vi "Periodic Tasks.vi"(11 "error in":errorcluster) -> ()   [LabVIEW 2012]
doc: "This VI runs in parallel to other tasks. It can contain as many user-defined periodic loops as you need. These can carry out PID or other sorts of timed response."
uses:
  <vilib>/Rock Robotics/SystemInterfaces/Utilities/FPGA_UtilitiesLED Source.ctl
  <vilib>/Rock Robotics/SystemInterfaces/Utilities/FPGA_UtilitiesLED State.ctl
  Global 1.vi
  Robot Global Data.vi
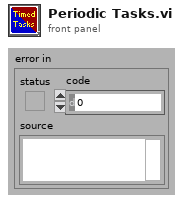
[diagram p1: front panel]
types:
  T1 = typedef "FPGA_UtilitiesLED State.ctl" = enum16{"Off", "On", "Toggle"}
  T2 = typedef "FPGA_UtilitiesLED Source.ctl" = enum16{"User LED", "FPGA LED"}
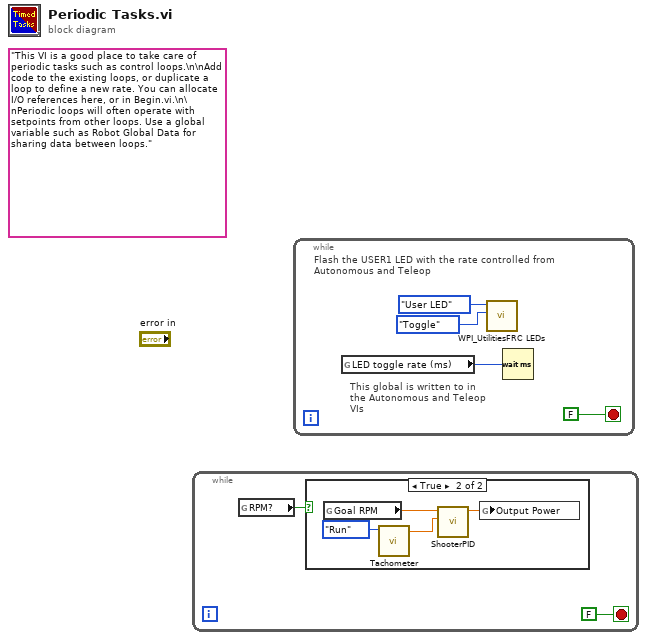
[diagram p0: block diagram]
diagram:
  (unwired) "This VI is a good place to take care of periodic tasks such as control loops.\n\nAdd code to the existing loops, or duplicate a loop to define a new rate. You can allocate I/O references here, or in Begin.vi.\n\nPeriodic loops will often operate with setpoints from other loops. Use a global variable such as Robot Global Data for sharing data between loops."
  n1 = while {
    stop <- FALSE stop-if-true
    n2 = global read "Global 1.vi" "RPM?"() -> (w2:bool)
    n3 = case shown="True" w2 {
      frame False {
      }
      frame True {
        n4 = global read "Global 1.vi" "Goal RPM"() -> (w6:dbl)
        n5 = call "Tachometer.vi"("Enum"=enum16{"Start", "Run", "End"}."Run") -> ("Tach out"=w4:dbl)  [unwired: 10 in]
        n6 = call "ShooterPID.vi"("Current"=w4, "Set"=w6) -> ("Shooter Motor"=w5:dbl)  [unwired: 9 in]
        n7 = global write "Global 1.vi" "Output Power"(w5) -> ()
      }
    }
  }
  n8 = while {
    stop <- FALSE stop-if-true
    # "This global is written to in the Autonomous and Teleop VIs"
    # "Flash the USER1 LED with the rate controlled from Autonomous and Teleop"
    n9 = global read "Robot Global Data.vi" "LED toggle rate (ms)"() -> (w7:u32)
    n10 = call <vilib>:"WPI_UtilitiesFRC LEDs.vi"("State"=FPGA_UtilitiesLED_State."Toggle", "LED Type"=FPGA_UtilitiesLED_Source."User LED") -> ()  [unwired: 1 in, 9 out]
    n11 = Wait (ms)(milliseconds to wait=w7) -> ()  [unwired: 1 out]
  }
